vi "Practica_2_Samael_Amado.vi"() -> ()   [LabVIEW 2021]
panel:
  in  "PARADA TOTAL":bool
  in  "ENCENDIDO / APAGADO":bool
  out "BANDA TRANSPORTADORA":bool
  out "MOTOR":bool
  out "CALDERA":bool
  out "VENTILADOR":bool
  # "TABLERO DE CONTROL"
  # "AREA DE TRABAJO"
  # "ACTIVIDAD INDIVIDUAL COMPONENTE PRÁCTICO 2\n\nSAMAEL AMADO HERNANDEZ\nSJAMADOH@UNADVIRTUAL.EDU.CO\nCC. 73240324\nTELEFONO: 3122987752\nGRUPO: 208055_1"
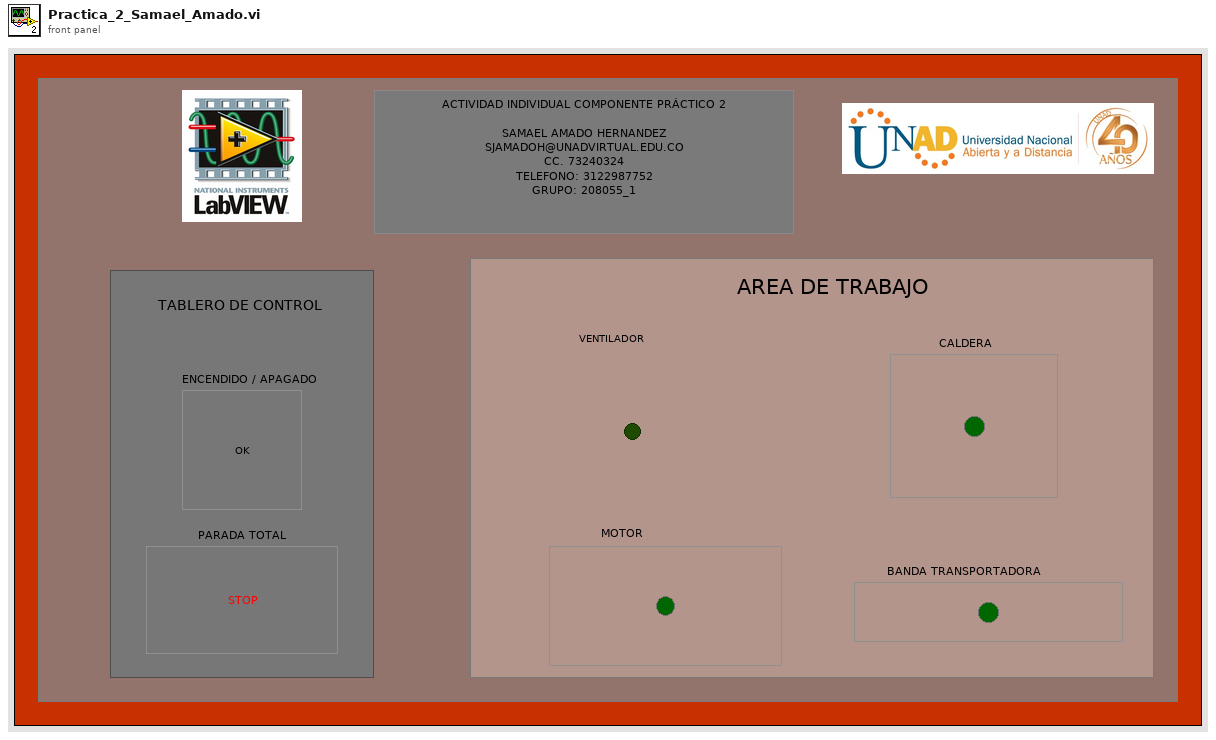
[diagram p1: front panel]
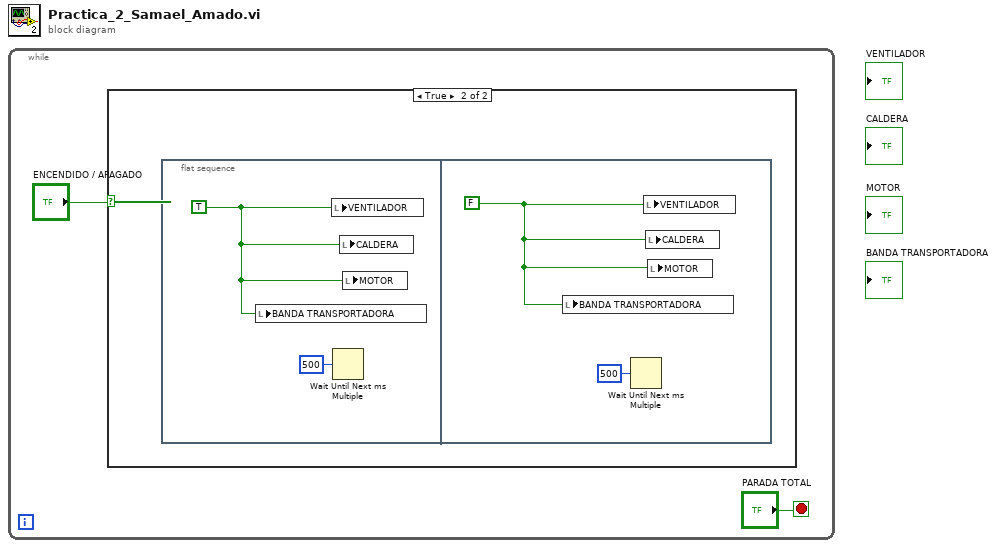
[diagram p0: block diagram]
diagram:
  n1 = while {
    stop <- "PARADA TOTAL" stop-if-true
    n2 = case shown="True" "ENCENDIDO / APAGADO" {
      frame False {
      }
      frame True {
        n3 = flat-sequence {
          frame #0 {
            w3 = TRUE ("Boolean")
            n4 = local write "BANDA TRANSPORTADORA"(w3) -> ()
            n5 = local write "VENTILADOR"(w3) -> ()
            n6 = Wait Until Next ms Multiple(millisecond multiple=u32 500) -> ()  [unwired: 1 out]
            n7 = local write "CALDERA"(w3) -> ()
            n8 = local write "MOTOR"(w3) -> ()
          }
          frame #1 {
            w5 = FALSE ("Boolean")
            n9 = local write "BANDA TRANSPORTADORA"(w5) -> ()
            n10 = Wait Until Next ms Multiple(millisecond multiple=u32 500) -> ()  [unwired: 1 out]
            n11 = local write "VENTILADOR"(w5) -> ()
            n12 = local write "CALDERA"(w5) -> ()
            n13 = local write "MOTOR"(w5) -> ()
          }
        }
      }
    }
  }
